vi "distributeHorizontalCenters.vi"(6 "useControlBodyOnly":bool, 7 "verticalAlignment":T1, 8 "error in (no error)":errorcluster, 11 "refs":refnum<vi>[](array[refnum])) -> (0 "error out":errorcluster, 3 "refs(dup)":refnum<vi>[](array[refnum]))   [LabVIEW 2023]
doc: "Arranges the input controls horizontally, making their centers equidistant. The leftmost and rightmost centers are kept fixed, while the other centers are distributed in between.\nThe vertical position is processed according to the input 'verticalArrangement'."
uses:
  Ctrls/alignment.ctl
  Misc/processUseControlBodyOnlyFlag_start.vi
  Misc/processUseControlBodyOnlyFlag_end.vi
  Misc/hideCaption&Label.vi
  Misc/setCaption&LabelVisibility.vi
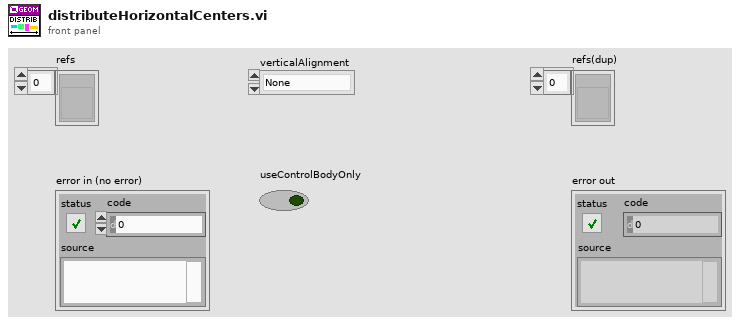
[diagram p1: front panel]
types:
  T1 = typedef "alignment.ctl" = enum16{"None", "AlignTop", "AlignBottom", "AlignHorizontalCenters", "AlignLeft", "AlignRight", "AlignVerticalCenters"}
  T2 = cluster{"horizontal":i32, "ref(dup)":refnum<vi>}[]
  T3 = cluster{"left":i32, "top":i32, "right":i32, "bottom":i32}
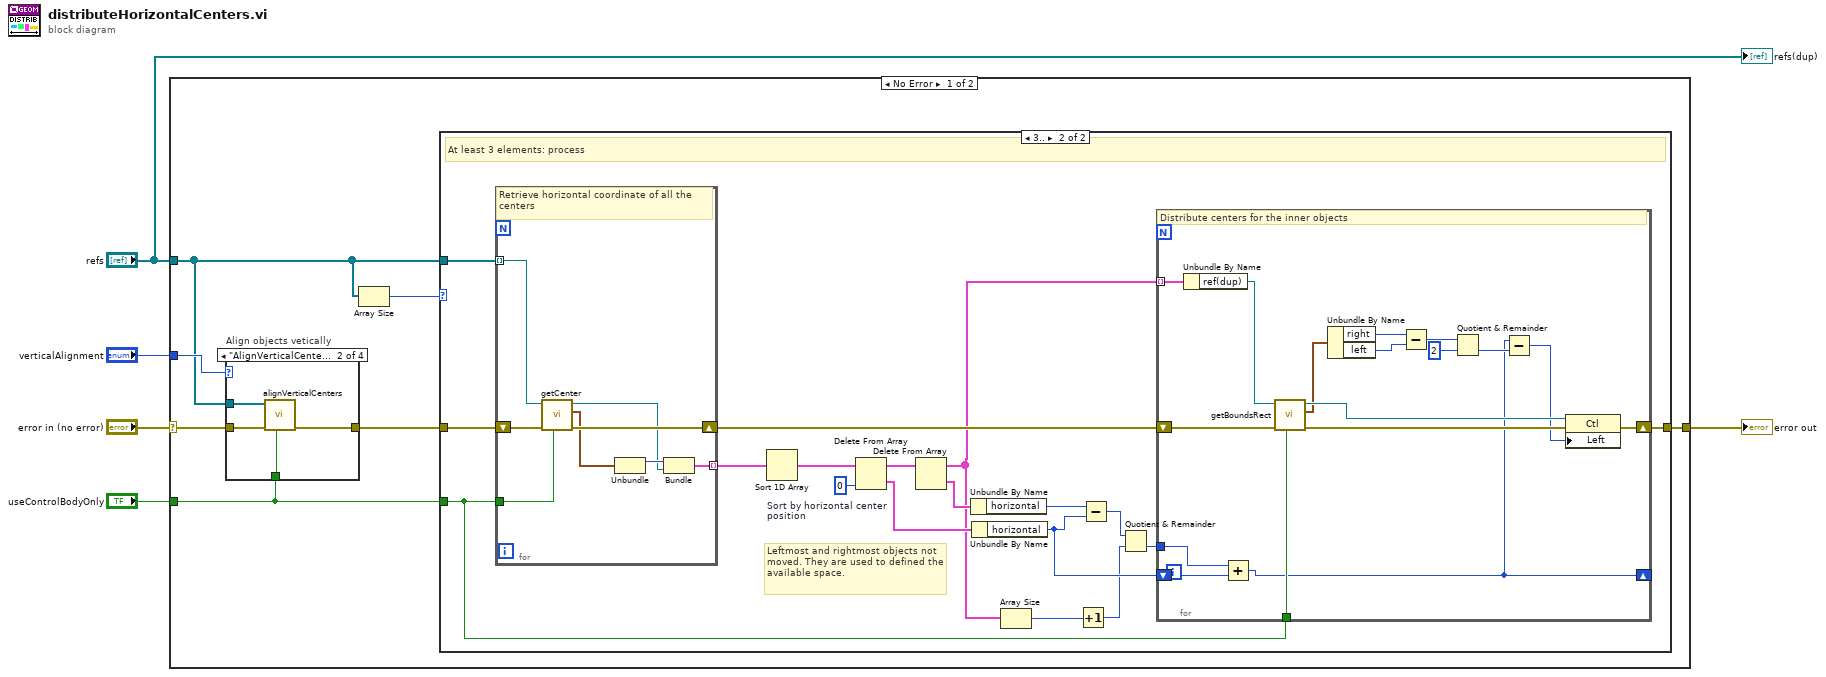
[diagram p0: block diagram]
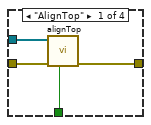
[diagram p3: hidden frame]
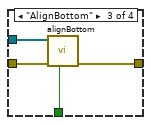
[diagram p4: hidden frame]
diagram:
  n1 = case shown="No Error" "error in (no error)" {
    selector: "error in (no error)" -> [w11 w70]
    tunnel: [w12 w70] -> w2
    tunnel: "refs" -> [w7 _]
    tunnel: "useControlBodyOnly" -> [w9 _]
    tunnel: "verticalAlignment" -> [w8 _]
    frame No Error {
      n2 = case "Align objects vetically" shown="\"AlignVerticalCenters\"" w8 {
        tunnel: w11 -> [w60 w64 w68 w69]
        tunnel: [w59 w63 w67 w69] -> w10
        tunnel: w9 -> [w58 w62 w66 _]
        tunnel: w7 -> [w57 w61 w65 _]
        frame "AlignTop" {
          n3 = call "alignTop.vi"("useControlBodyOnly"=w58, "error in (no error)"=w60, "refs"=w57) -> ("error out"=w59:errorcluster)  [unwired: 7 in, 1 out]
        }
        frame "AlignVerticalCenters" {
          n4 = call "alignVerticalCenters.vi"("useControlBodyOnly"=w62, "error in (no error)"=w64, "refs"=w61) -> ("error out"=w63:errorcluster)  [unwired: 7 in, 1 out]
        }
        frame "AlignBottom" {
          n5 = call "alignBottom.vi"("useControlBodyOnly"=w66, "error in (no error)"=w68, "refs"=w65) -> ("error out"=w67:errorcluster)  [unwired: 7 in, 1 out]
        }
        frame "None", Default {
        }
      }
      n6 = Array Size(array=w7) -> (size(s)=w6:i32)
      n7 = case shown="3.." w6 {
        tunnel: [w13 w21] -> w12
        tunnel: w10 -> [w13 w31]
        tunnel: w9 -> [_ w20]
        tunnel: w7 -> [_ w30]
        frame ..2 {
          # "Not enough elements: do nothing"
        }
        frame 3.. {
          # "Leftmost and rightmost objects not moved. They are used to defined the available space."
          # "At least 3 elements: process"
          n8 = for {
            shift-right: [w55] -> w22
            shift-left: w31 -> [w56]
            tunnel: w30 -> [w53] mode=indexing
            tunnel: w20 -> [w54]
            tunnel: [w49] -> w29 mode=indexing
            # "Retrieve horizontal coordinate of all the centers"
            n9 = call "getCenter.vi"("useControlBodyOnly"=w54, "error in (no error)"=w56, "ref"=w53) -> ("error out"=w55:errorcluster, "center"=w52:cluster{"horizontal":i32, "vertical":i32}, "ref(dup)"=w50:refnum<vi>)  [unwired: 6 in]
            n10 = Unbundle(w52) -> ("horizontal"=w51:i32)  [unwired: 1 out]
            n11 = Bundle("horizontal"=w51, "ref(dup)"=w50) -> (w49:cluster{"horizontal":i32, "ref(dup)":refnum<vi>})  [unwired: 1 in]
          }
          n12 = Sort 1D Array "Sort by horizontal center position"(array=w29) -> (sorted array=w17:T2)
          n13 = Delete From Array(array=w17, index=0) -> (deleted portion=w25:cluster{"horizontal":i32, "ref(dup)":refnum<vi>}, array with subset deleted=w27:T2)  [unwired: 1 in]
          n14 = Delete From Array(array=w27) -> (deleted portion=w26:cluster{"horizontal":i32, "ref(dup)":refnum<vi>}, array with subset deleted=w16:T2)  [unwired: 2 in]
          n15 = Unbundle By Name(w26) -> ("horizontal"=w24:i32)
          n16 = Unbundle By Name(w25) -> ("horizontal"=w18:i32)
          n17 = Array Size(array=w16) -> (size(s)=w15:i32)
          n18 = Increment(x=w15) -> (x+1=w14:i32)
          n19 = Subtract(x=w24, y=w18) -> (x-y=w23:i32)
          n20 = Quotient & Remainder(x=w23, y=w14) -> (floor(x/y)=w19:i32)  [unwired: 1 out]
          n21 = for {
            shift-right: [w37] -> w21
            shift-left: w22 -> [w38]
            tunnel: w19 -> [w33]
            tunnel: w16 -> [w48] mode=indexing
            tunnel: w20 -> [w35]
            shift-right: [w32] -> _
            shift-left: w18 -> [w34]
            # "Distribute centers for the inner objects"
            n22 = Unbundle By Name(w48) -> ("ref(dup)"=w36:refnum<vi>)
            n23 = Add(x=w33, y=w34) -> (x+y=w32:i32)
            n24 = call "getBoundsRect.vi"("useControlBodyOnly"=w35, "error in (no error)"=w38, "ref"=w36) -> ("error out"=w43:errorcluster, "rect"=w41:T3, "ref(dup)"=w42:refnum<vi>)  [unwired: 6 in]
            n25 = Unbundle By Name(w41) -> ("right"=w47:i32, "left"=w46:i32)
            n26 = Subtract(x=w47, y=w46) -> (x-y=w44:i32)
            n27 = Quotient & Remainder(x=w44, y=2) -> (floor(x/y)=w45:i32)  [unwired: 1 out]
            n28 = Subtract(x=w32, y=w45) -> (x-y=w39:i32)
            n29 = property class="Ctl"(reference=w42, error in=w43, "Left"=w39) -> (error out=w37:errorcluster)  [unwired: 1 out]
          }
        }
      }
    }
    frame Error {
    }
  }
  "error out" <- w2
  "refs(dup)" <- "refs"
